vi "AnalogWaveformProbe_CXT_phase_deg.vi"(1 "Waveform":waveform(cxt)={"t0"=timestamp(0 s since 1904-01-01), "dt"=0.0, "Y"=[]}) -> (0 "Stop if?":bool)   [LabVIEW 2017]
doc: "Displays a graph of the analog data; a table with a time stamp that specifies when the probe received the data, the x value, and the time; and a table that displays the attributes of the waveform data type."
uses:
  <vilib>/Utility/error.llb/ErrWarn.ctl
panel:
  in  "x":string="x"
  in  "t":string="t"
  in  "Tab Control":T1(tab)
  out "Timestamp":timestamp format="%<%X\n%x>T"
  out "Waveform Graph":waveform(dbl)(graph) caption="Waveform Graph 2"
  in  "warn icon":T2
  in  "warning msg":string="Table data truncated to\nlimit memory usage."
  out "Start t":timestamp format="%<%X\n%x>T"
  out "Data":string[][](table)
  out "Attributes":variant
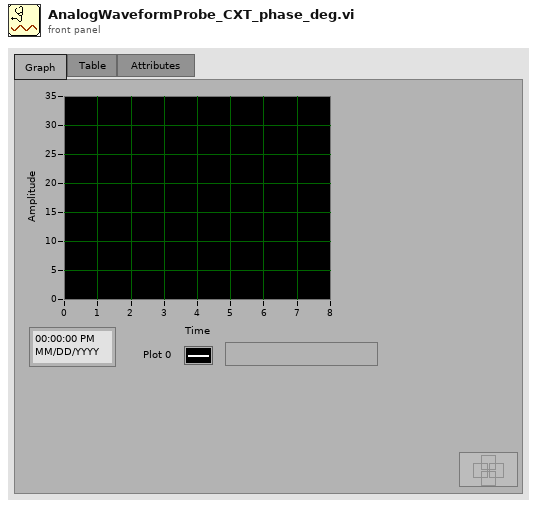
[diagram p1: front panel]
types:
  T1 = enum32{"Graph   ", "Table   ", "Attributes     "}
  T2 = typedef "ErrWarn.ctl" = bool
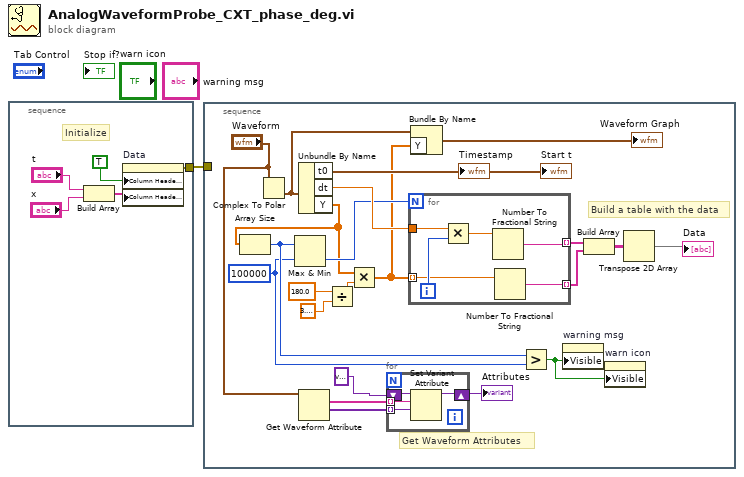
[diagram p0: block diagram]
diagram:
  n1 = stacked-sequence {
    tunnel: [w2] -> w1
    frame #0 {
      # "Initialize"
      n2 = Build Array("t", "x") -> (w4:string[])
      n3 = property on="Data" class="Tbl (strict)"("Column Headers Visible"=TRUE, "Column Header Strings[]"=w4) -> (error out=w2:errorcluster)  [unwired: 2 in, 1 out]
    }
  }
  n4 = stacked-sequence {
    tunnel: w1 -> [_]
    frame #0 {
      w16 = 100000
      # "Get Waveform Attributes"
      # "Build a table with the data"
      n5 = Complex To Polar(r * e^(i*theta)="Waveform") -> (theta=w9:waveform(dbl))  [unwired: 1 out]
      n6 = Unbundle By Name(w9) -> ("t0"=→"Timestamp" →"Start t":timestamp, "dt"=w28:dbl, "Y"=w11:dbl[])
      n7 = Array Size(array=w11) -> (size(s)=w17:i32)
      n8 = Max & Min(x=w17, y=w16) -> (min(x,y)=w18:i32)  [unwired: 1 out]
      n9 = Get Waveform Attribute(7:"Waveform") -> (1:w21:variant[], 2:w22:string[])  [unwired: 3 in, 2 out]
      n10 = Divide(x=180.0, y=3.141592653589793) -> (x/y=w12:dbl)
      n11 = Multiply(x=w11, y=w12) -> (x*y=w8:dbl[])
      n12 = for {
        tunnel: w22 -> [w31] mode=indexing
        tunnel: w21 -> [w32] mode=indexing
        shift-right: [w29] -> w19
        shift-left: variant ("variant") -> [w30]
        n13 = Set Variant Attribute(Variant=w30, name=w31, value=w32) -> (Variant out=w29:variant)  [unwired: 1 in, 2 out]
      }
      "Attributes" <- w19
      n14 = for {
        N: w18 -> [_]
        tunnel: [w36] -> w25 mode=indexing
        tunnel: w8 -> [w35] mode=indexing
        tunnel: w28 -> [w38]
        tunnel: [w33] -> w24 mode=indexing
        i -> [w37]
        n15 = Multiply(x=w38, y=w37) -> (x*y=w34:dbl)
        n16 = Number To Fractional String(number=w34) -> (F-format string=w33:string)  [unwired: 3 in]
        n17 = Number To Fractional String(number=w35) -> (F-format string=w36:string)  [unwired: 3 in]
      }
      n18 = Bundle By Name(cluster=w9, "Y"=w8) -> (→"Waveform Graph":waveform(dbl))
      n19 = Greater?(x=w17, y=w16) -> (0:w15:bool)
      n20 = property on="warning msg" class="Str"("Visible"=w15) -> ()  [unwired: 2 in, 2 out]
      n21 = Build Array(w24, w25) -> (w27:string[][])
      n22 = property on="warn icon" class="Bool"("Visible"=w15) -> ()  [unwired: 2 in, 2 out]
      n23 = Transpose 2D Array(2D array=w27) -> (transposed array=→"Data":string[][])
    }
  }
